vi "Main.vi"() -> ()   [LabVIEW 2022 SP3]
uses:
  MusicPlayer_class/MusicPlayer.lvclass
panel:
  out "Current Song":string
  in  "Add":bool
  in  "Exit":bool
  in  "Clear":bool
  in  "Remove":bool
  in  "Previous":bool
  in  "Next":bool
  in  "Playlist":i32(listbox)
  in  "Stop":bool
  in  "Play":bool
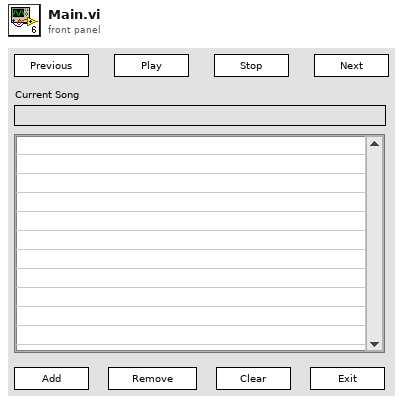
[diagram p1: front panel]
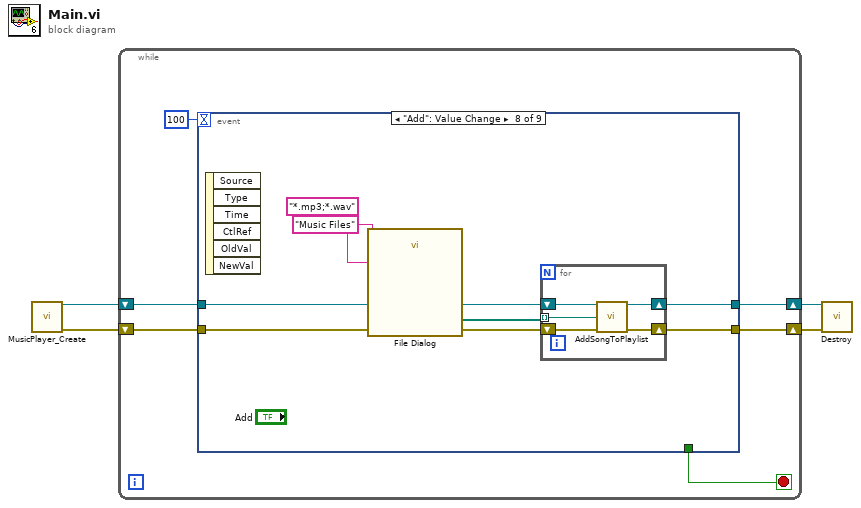
[diagram p0: block diagram]
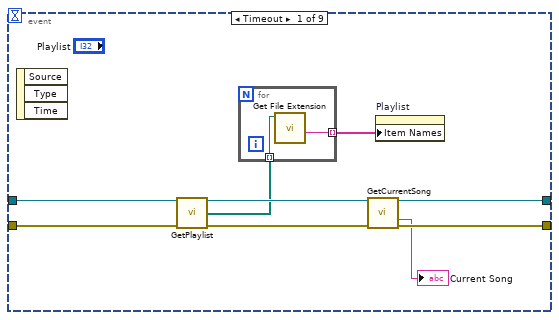
[diagram p2: hidden frame]
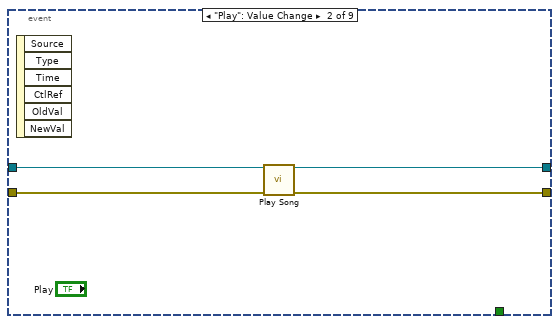
[diagram p3: hidden frame]
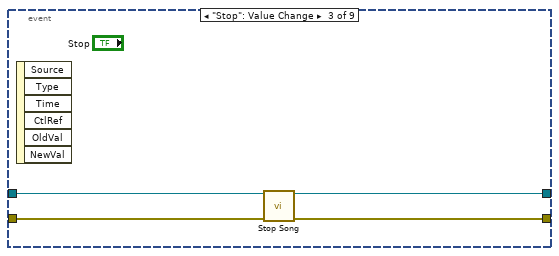
[diagram p4: hidden frame]
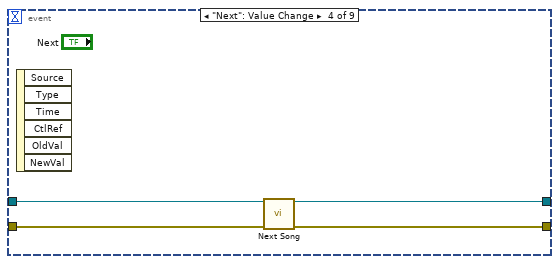
[diagram p5: hidden frame]
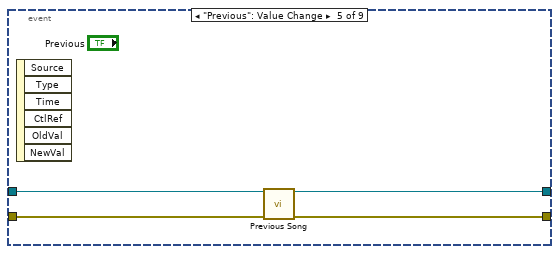
[diagram p6: hidden frame]
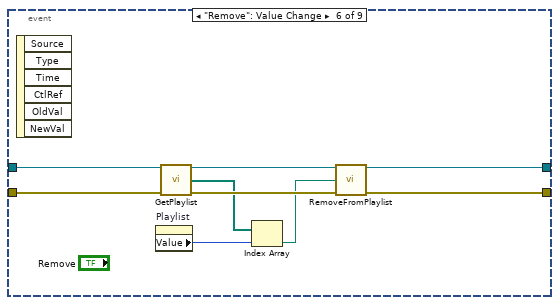
[diagram p7: hidden frame]
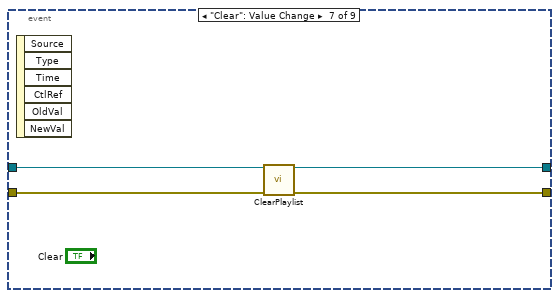
[diagram p8: hidden frame]
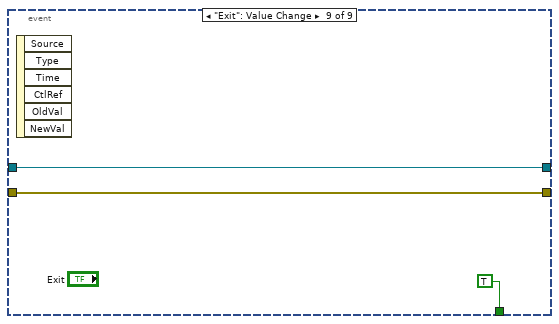
[diagram p9: hidden frame]
diagram:
  n1 = call "MusicPlayer_Create.vi"() -> ("reference out"=w3:refnum<class "MusicPlayer.lvclass">, "Error Out"=w4:errorcluster)  [unwired: 14 in]
  n2 = while {
    shift-right: [w7] -> w1
    shift-left: w4 -> [w8]
    shift-right: [w6] -> w2
    shift-left: w3 -> [w5]
    stop <- w10 stop-if-true
    n3 = event shown="[7] \"Add\": Value Change" {
      selector: _ -> [_ _ _ _ _ _ _ _ _]
      dyn-events: _ -> [_ _ _ _ _ _ _ _ _]
      timeout: 100 -> [_ _ _ _ _ _ _ _ _]
      tunnel: [_ _ _ _ _ _ _ _ TRUE] -> w10
      tunnel: w8 -> [w19 w25 w29 w33 w37 w46 w50 w51 w65]
      tunnel: [w18 w24 w28 w32 w36 w45 w49 w58 w65] -> w7
      tunnel: w5 -> [w14 w23 w27 w31 w35 w42 w48 w57 w64]
      tunnel: [w17 w22 w26 w30 w34 w44 w47 w56 w64] -> w6
      event Timeout {
        n4 = event-data() -> ()  [unwired: 1 in, 3 out]
        n5 = call "GetPlaylist.vi"("reference in"=w14, "Error In"=w19) -> ("reference out"=w13:refnum<class "MusicPlayer.lvclass">, "Playlist"=w12:path[], "Error Out"=w15:errorcluster)  [unwired: 11 in]
        n6 = for {
          tunnel: w12 -> [w21] mode=indexing
          tunnel: [w20] -> w11 mode=indexing
          n7 = call <vilib>:"Get File Extension.vi"("file"=w21) -> ("filename without extension"=w20:string)  [unwired: 6 in, 4 out]
        }
        n8 = call-dynamic "GetCurrentSong.vi"("reference in"=w13, "Error In"=w15) -> ("reference out"=w17:refnum<class "MusicPlayer.lvclass">, "Song Name"=→"Current Song":string, "Error Out"=w18:errorcluster)  [unwired: 10 in, 1 out]
        n9 = property on="Playlist" class="LstBox (strict)"("Item Names"=w11) -> ()  [unwired: 2 in, 2 out]
      }
      event "Play": Value Change {
        n10 = event-data() -> ()  [unwired: 1 in, 6 out]
        n11 = call-dynamic "Play Song.vi"("reference in"=w23, "Error In"=w25) -> ("reference out"=w22:refnum<class "MusicPlayer.lvclass">, "Error Out"=w24:errorcluster)  [unwired: 12 in]
      }
      event "Stop": Value Change {
        n12 = event-data() -> ()  [unwired: 1 in, 6 out]
        n13 = call-dynamic "Stop Song.vi"("reference in"=w27, "Error In"=w29) -> ("reference out"=w26:refnum<class "MusicPlayer.lvclass">, "Error Out"=w28:errorcluster)  [unwired: 12 in]
      }
      event "Next": Value Change {
        n14 = event-data() -> ()  [unwired: 1 in, 6 out]
        n15 = call-dynamic "Next Song.vi"("reference in"=w31, "Error In"=w33) -> ("reference out"=w30:refnum<class "MusicPlayer.lvclass">, "Error Out"=w32:errorcluster)  [unwired: 12 in]
      }
      event "Previous": Value Change {
        n16 = event-data() -> ()  [unwired: 1 in, 6 out]
        n17 = call-dynamic "Previous Song.vi"("reference in"=w35, "Error In"=w37) -> ("reference out"=w34:refnum<class "MusicPlayer.lvclass">, "Error Out"=w36:errorcluster)  [unwired: 12 in]
      }
      event "Remove": Value Change {
        n18 = event-data() -> ()  [unwired: 1 in, 6 out]
        n19 = property on="Playlist" class="LstBox (strict)"() -> ("Value"=w39:i32)  [unwired: 2 in, 2 out]
        n20 = call "GetPlaylist.vi"("reference in"=w42, "Error In"=w46) -> ("reference out"=w41:refnum<class "MusicPlayer.lvclass">, "Playlist"=w40:path[], "Error Out"=w43:errorcluster)  [unwired: 11 in]
        n21 = Index Array(array=w40, index=w39) -> (element=w38:path)
        n22 = call-dynamic "RemoveFromPlaylist.vi"("reference in"=w41, "File Path"=w38, "Error In"=w43) -> ("reference out"=w44:refnum<class "MusicPlayer.lvclass">, "Error Out"=w45:errorcluster)  [unwired: 11 in]
      }
      event "Clear": Value Change {
        n23 = event-data() -> ()  [unwired: 1 in, 6 out]
        n24 = call-dynamic "ClearPlaylist.vi"("reference in"=w48, "Error In"=w50) -> ("reference out"=w47:refnum<class "MusicPlayer.lvclass">, "Error Out"=w49:errorcluster)  [unwired: 12 in]
      }
      event "Add": Value Change {
        n25 = event-data() -> ()  [unwired: 1 in, 6 out]
        n26 = call "File Dialog"("error in"=w51, "pattern (all files)"="*.mp3;*.wav", "pattern label"="Music Files") -> ("selected paths"=w53:path[], "error out"=w52:errorcluster)  [unwired: 9 in, 2 out]
        n27 = for {
          shift-right: [w62] -> w58
          shift-left: w52 -> [w63]
          shift-right: [w60] -> w56
          shift-left: w57 -> [w61]
          tunnel: w53 -> [w59] mode=indexing
          n28 = call-dynamic "AddSongToPlaylist.vi"("reference in"=w61, "File Path"=w59, "Error In"=w63) -> ("reference out"=w60:refnum<class "MusicPlayer.lvclass">, "Error Out"=w62:errorcluster)  [unwired: 11 in]
        }
      }
      event "Exit": Value Change {
        n29 = event-data() -> ()  [unwired: 1 in, 6 out]
      }
    }
  }
  n30 = call-dynamic "Destroy.vi"("reference in"=w2, "Error In"=w1) -> ()  [unwired: 12 in, 2 out]
